vi "TextTestRunner.JUnitXML_Init.vi"(8 "error in (no error)":errorcluster, 9 "Report Path":path, 11 "TextTestRunner in":refnum<class "TextTestRunner.JUnitXML.lvclass">) -> (0 "error out":errorcluster, 3 "TextTestRunner out":refnum<class "TextTestRunner.JUnitXML.lvclass">)   [LabVIEW 2011, in "TextTestRunner.JUnitXML.lvclass"]
uses:
  TextTestRunner.JUnitXML.lvclass
  TextTestRunner.JUnitXML.lvclass/TextTestRunner.JUnitXML.ctl
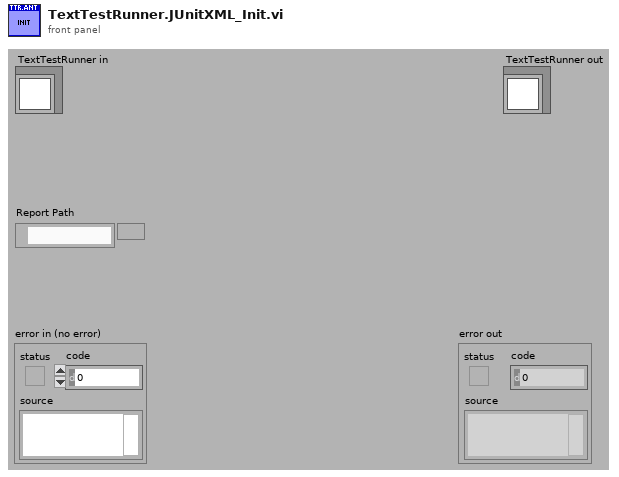
[diagram p1: front panel]
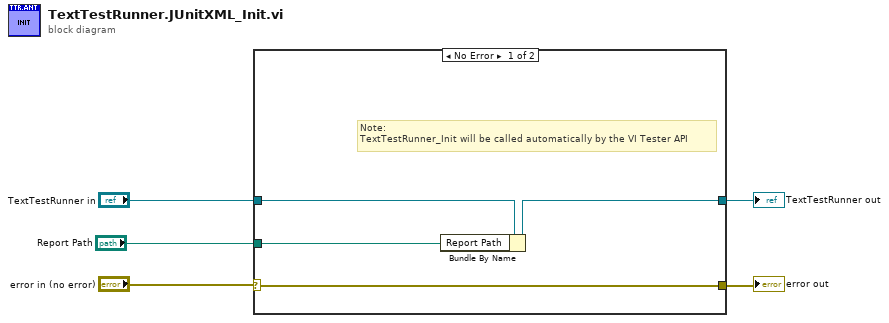
[diagram p0: block diagram]
diagram:
  n1 = case shown="No Error" "error in (no error)" {
    selector: "error in (no error)" -> [w6 w10]
    tunnel: "TextTestRunner in" -> [w9 w11]
    tunnel: [w7 w11] -> w4
    tunnel: [w6 w10] -> w2
    tunnel: "Report Path" -> [w8 _]
    frame No Error {
      # "Note:\nTextTestRunner_Init will be called automatically by the VI Tester API"
      n2 = Bundle By Name(cluster=w9, "Report Path"=w8) -> (w7:refnum<class "TextTestRunner.JUnitXML.lvclass">)
    }
    frame Error {
    }
  }
  "TextTestRunner out" <- w4
  "error out" <- w2
